vi "RANGE.vi"(8 "error in (no error)":errorcluster, 11 "range_str":string) -> (0 "error out":errorcluster, 1 "row2":u32, 2 "col":u16, 3 "row":u32, 5 "col2":u16)   [LabVIEW 8.6]
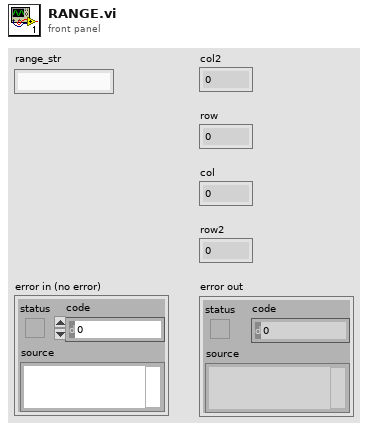
[diagram p1: front panel]
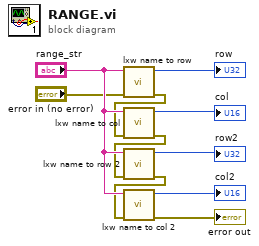
[diagram p0: block diagram]
diagram:
  n1 = call "lxw name to row.vi"("error in (no error)"="error in (no error)", "row_str"="range_str") -> ("error out"=w1:errorcluster, "function return"=→"row":u32)  [unwired: 8 in]
  n2 = call "lxw name to col.vi"("error in (no error)"=w1, "col_str"="range_str") -> ("error out"=w2:errorcluster, "function return"=→"col":u16)  [unwired: 8 in]
  n3 = call "lxw name to row 2.vi"("error in (no error)"=w2, "row_str"="range_str") -> ("error out"=w3:errorcluster, "function return"=→"row2":u32)  [unwired: 8 in]
  n4 = call "lxw name to col 2.vi"("error in (no error)"=w3, "col_str"="range_str") -> ("error out"=→"error out":errorcluster, "function return"=→"col2":u16)  [unwired: 8 in]
